vi "D-Lockin.vi"(8 "error in (no error)":errorcluster, 9 "index":u32, 10 "Stop?":bool, 11 "SweepControl":refnum<class "SMO.SweepControl.lvclass">) -> (0 "error out":errorcluster, 3 "SweepControl":refnum<class "SMO.SweepControl.lvclass">)   [LabVIEW 2019, in "SMO.SweepControl.lvclass"]
uses:
  SMO.SweepControl.lvclass
  <userlib>/LevyLab/Lockin-Multichannel/Instrument.Lockin/Instrument.Lockin.lvclass
  SMO.Transport/SMO.Transport.lvclass
  Control Experiment/Control Experiment.lvclass
  <userlib>/LevyLab/Lockin-Multichannel/Instrument.Lockin/Typedefs/Results Type--Enum.ctl
  SMO.Control Experiment/SMO.Control Experiment.lvclass
  C:/Program Files (x86)/National Instruments/LabVIEW 2019/user.lib/LevyLab/Instrument Framework/SMOs/Instrument/Instrument.lvclass
  C:/Program Files (x86)/National Instruments/LabVIEW 2019/vi.lib/JKI/JKI SMO/SMO/SMO.lvclass
panel:
  out "G4T":cluster{dbl[], dbl[]}[](graph)
  out "Y Lockins":cluster{dbl[], dbl[]}[](graph)
  out "X Lockins":cluster{dbl[], dbl[]}[](graph)
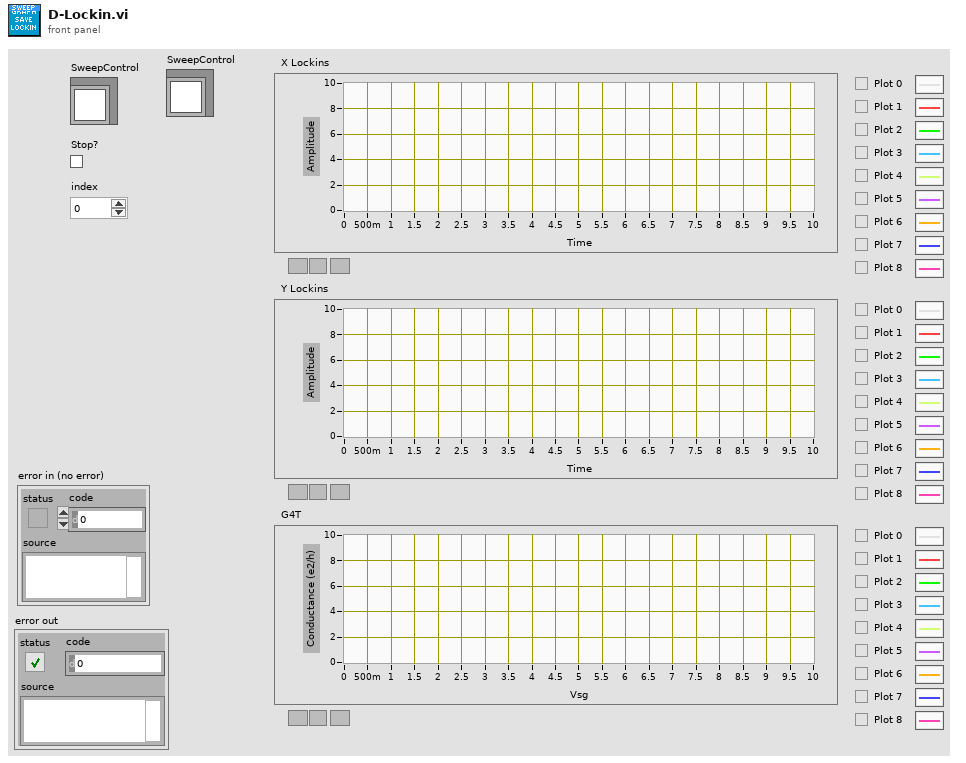
[diagram p1: front panel]
types:
  T1 = cluster{"Result X":dbl[], "Result Y":dbl[], "Data":cluster{"Y  Array":dbl[]}[], "wavenames":string[], "All Result X":dbl[][], "All Result Y":dbl[][]}
  T2 = cluster{"SweepControl":refnum<class "SMO.SweepControl.lvclass">, "data":cluster{"Result X":dbl[], "Result Y":dbl[], "Data":cluster{"Y  Array":dbl[]}[], "wavenames":string[], "All Result X":dbl[][], "All Result Y":dbl[][]}, "All Parameters":dbl[]}
  T3 = typedef "Instrument.Lockin.lvclass/Results Type--Enum.ctl" = enum16{"X", "Y", "R", "Theta", "Mean"}
  T4 = typedef "Control Experiment.lvclass/Instruments--cluster.ctl" = cluster{"KH7008":refnum<class "Instrument.KH7008.lvclass">[], "Lockin":refnum<class "Instrument.Lockin.lvclass">, "Temperature":refnum<class "Instrument.Cryostat.lvclass">, "Magnet":refnum<class "Instrument.Cryostat.lvclass">, "Rotator":refnum<class "Instrument.Cryostat.lvclass">, "Level":refnum<class "Instrument.Cryostat.lvclass">, "Capacitance Bridge":refnum<class "Instrument.CBridge.lvclass">, "Delay Line":refnum<class "Instrument.DelayLine.lvclass">, "Strain Cell":refnum<class "Instrument.Strain.lvclass">, "VNA":refnum<class "Instrument.VNA.lvclass">, "Voltage Source":refnum<class "Instrument.VSource.lvclass">}
  T5 = cluster{"I-":i32, "I+":i32, "V1-":i32, "V1+":i32, "I2-":i32, "I2+":i32, "V2-":i32, "V2+":i32}
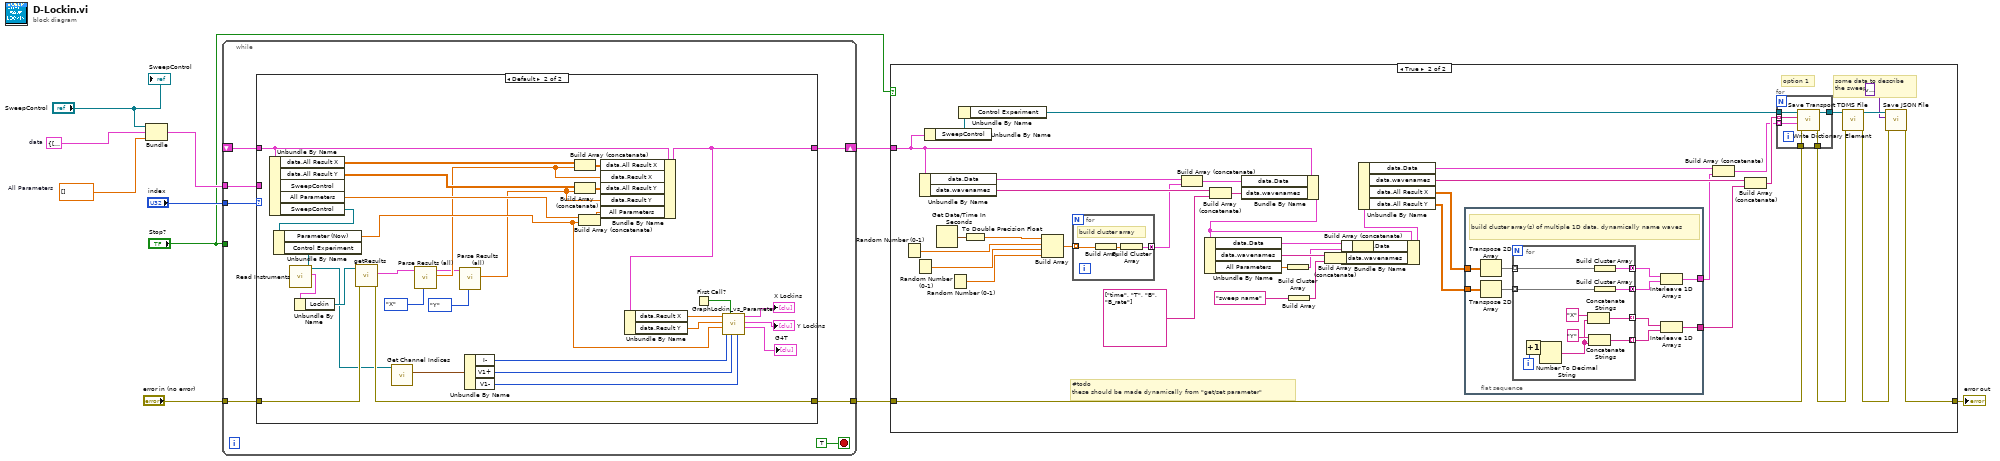
[diagram p0: block diagram]
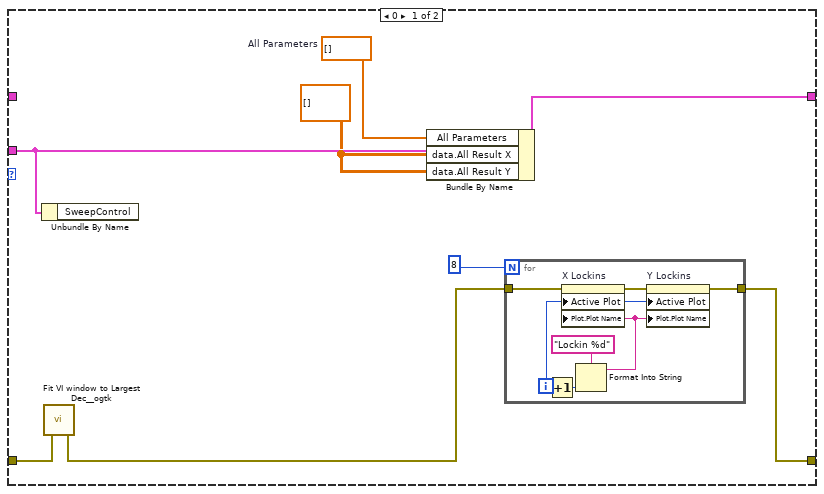
[diagram p3: hidden frame]
diagram:
  w3 = dbl[] []  # All Parameters
  w6 = T1 {"Result X"=[], "Result Y"=[], "Data"=[], "wavenames"=[], "All Result X"=[], "All Result Y"=[]}  # data
  n1 = Bundle("SweepControl"="SweepControl", "data"=w6, "All Parameters"=w3) -> (w7:T2)  [unwired: 1 in]
  n2 = while {
    tunnel: "index" -> [w17]
    tunnel: "Stop?" -> [_]
    tunnel: "error in (no error)" -> [w16]
    shift-right: [w14] -> w4
    shift-left: _ -> [w15]
    tunnel: w7 -> [w13]
    tunnel: [w12] -> w2
    stop <- TRUE stop-if-true
    n3 = case shown="Default" w17 {
      tunnel: w16 -> [w21 w60]
      tunnel: w15 -> [_ w58]
      tunnel: [w25 w56] -> w14
      tunnel: w13 -> [w24 _]
      tunnel: [w22 w59] -> w12
      frame 0 {
        w19 = dbl[] []  # All Parameters
        w20 = dbl[][] [] ("data.All Result X")
        n4 = Unbundle By Name(w24) -> ()  [unwired: 1 out]
        n5 = call <userlib>:"Fit VI window to Largest Dec__ogtk.vi"("error in (no error)"=w21) -> ("error out"=w18:errorcluster)  [unwired: 5 in, 1 out]
        n6 = Bundle By Name(cluster=w24, "All Parameters"=w19, "data.All Result X"=w20, "data.All Result Y"=w20) -> (w25:T2)
        n7 = for {
          N: 8 -> [_]
          tunnel: [w27] -> w22
          tunnel: w18 -> [w26]
          i -> [w30]
          n8 = Increment(x=w30) -> (x+1=w28:i32)
          n9 = Format Into String(format string="Lockin %d", w28) -> (resulting string=w31:string)  [unwired: 2 in, 1 out]
          n10 = property on="X Lockins" class="XYGraph (strict)"(error in=w26, "Active Plot"=w30, "Plot.Plot Name"=w31) -> (error out=w29:errorcluster)  [unwired: 1 in, 1 out]
          n11 = property on="Y Lockins" class="XYGraph (strict)"(error in=w29, "Active Plot"=w30, "Plot.Plot Name"=w31) -> (error out=w27:errorcluster)  [unwired: 1 in, 1 out]
        }
      }
      frame Default {
        n12 = Unbundle By Name(w58) -> ("data.All Result X"=w64:dbl[][], "data.All Result Y"=w63:dbl[][], "All Parameters"=w53:dbl[], "SweepControl"=w52:refnum<class "SMO.SweepControl.lvclass">)  [unwired: 1 out]
        n13 = Unbundle By Name(w52) -> ("Parameter (Now)"=w51:dbl, "Control Experiment"=w46:refnum<class "SMO.Control Experiment.lvclass">)
        n14 = call "Read Instruments.vi"("Control Experiment in"=w46) -> ("Instruments"=w45:T4, "Control Experiment out"=w43:refnum<class "Control Experiment.lvclass">)  [unwired: 8 in, 1 out]
        n15 = Unbundle By Name(w45) -> ("Lockin"=w44:refnum<class "Instrument.Lockin.lvclass">)
        n16 = call <userlib>:"getResults.vi"("error in (no error)"=w60, "Instrument.Lockin in"=w44) -> ("error out"=w59:errorcluster, "Results (Dictionary)"=w38:cluster{"key":string, "value":dbl}[])  [unwired: 6 in, 2 out]
        n17 = call "Get Channel Indices.vi"("Control Experiment in"=w43) -> ("Indices"=w42:T5)  [unwired: 8 in, 2 out]
        n18 = call <userlib>:"Parse Results (all).vi"("Type"=Results_Type--Enum."X", "Results (Dictionary)"=w38) -> ("Data"=w37:dbl[], "Results (Dictionary)"=w35:cluster{"key":string, "value":dbl}[])  [unwired: 6 in, 2 out]
        n19 = call <userlib>:"Parse Results (all).vi"("Type"=Results_Type--Enum."Y", "Results (Dictionary)"=w35) -> ("Data"=w36:dbl[])  [unwired: 6 in, 3 out]
        n20 = Unbundle By Name(w42) -> ("I-"=w41:i32, "V1+"=w40:i32, "V1-"=w39:i32)
        n21 = Build Array (concatenate)(w64, w37) -> (w61:dbl[][])
        n22 = Build Array (concatenate)(w63, w36) -> (w62:dbl[][])
        n23 = Build Array (concatenate)(w53, w51) -> (w50:dbl[])
        n24 = Bundle By Name(cluster=w58, "data.All Result X"=w61, "data.Result X"=w37, "data.All Result Y"=w62, "data.Result Y"=w36, "All Parameters"=w50) -> (w56:T2)
        n25 = Unbundle By Name(w56) -> ("data.Result X"=w57:dbl[], "data.Result Y"=w54:dbl[])
        n26 = First Call?() -> (First Call?: T/F=w55:bool)
        n27 = call "GraphLockin_vs_Parameter.vi"("V-"=w39, "V+"=w40, "reset?"=w55, "Current"=w41, "Parameter"=w51, "Y[ ]"=w54, "X[ ]"=w57) -> ("G(e2/h) vs Parameter"=→"G4T":cluster{"Y":dbl[], "Y":dbl[]}[], "Y vs Parameter"=→"Y Lockins":cluster{dbl[], dbl[]}[], "X vs Parameter"=→"X Lockins":cluster{dbl[], dbl[]}[])  [unwired: 1 in, 1 out]
      }
    }
  }
  n28 = case shown="True" "Stop?" {
    tunnel: w4 -> [_ w79]
    tunnel: w2 -> [w65 w67]
    tunnel: [w65 w73] -> w1
    frame False {
    }
    frame True {
      # "option 1"
      # "some data to describe\nthe sweep"
      # "#todo\nthese should be made dynamically from \"get/set parameter\""
      n29 = Random Number (0-1)() -> (number: 0 to 1=w96:dbl)
      n30 = Random Number (0-1)() -> (number: 0 to 1=w95:dbl)
      n31 = Unbundle By Name(w79) -> ("data.Data"=w105:cluster{"Y  Array":dbl[]}[], "data.wavenames"=w104:string[])
      n32 = Unbundle By Name(w79) -> ("SweepControl"=w78:refnum<class "SMO.SweepControl.lvclass">)
      n33 = Get Date/Time In Seconds() -> (seconds since 1Jan1904=w100:timestamp)
      n34 = Random Number (0-1)() -> (number: 0 to 1=w94:dbl)
      n35 = Unbundle By Name(w78) -> ("Control Experiment"=w68:refnum<class "SMO.Control Experiment.lvclass">)
      n36 = To Double Precision Float(number=w100) -> (double precision float=w99:dbl)
      n37 = Build Array(w99, w96, w95, w94) -> (w97:dbl[])
      n38 = for {
        tunnel: [w134] -> w98 mode=concatenating
        tunnel: w97 -> [w133] mode=indexing
        # "build cluster array"
        n39 = Build Array(w133) -> (w135:dbl[])
        n40 = Build Cluster Array(w135) -> (w134:cluster{dbl[]}[])
      }
      n41 = Build Array (concatenate)(w105, w98) -> (w102:cluster{"Y  Array":dbl[]}[])
      n42 = Build Array (concatenate)(w104, string[] ["time", "T", "B", "B_rate"] ("wavenames (.Vx, etc)")) -> (w103:string[])
      n43 = Bundle By Name(cluster=w79, "data.Data"=w102, "data.wavenames"=w103) -> (w81:T2)
      n44 = Unbundle By Name(w81) -> ("data.Data"=w93:cluster{"Y  Array":dbl[]}[], "data.wavenames"=w92:string[], "All Parameters"=w90:dbl[])
      n45 = Build Cluster Array(w90) -> (w89:cluster{"All Parameters":dbl[]}[])
      n46 = Build Array("sweep name" ("wavenames")) -> (w86:string[])
      n47 = Build Array (concatenate)(w92, w86) -> (w88:string[])
      n48 = Build Array (concatenate)(w93, w89) -> (w91:cluster{"All Parameters":dbl[]}[])
      n49 = Bundle By Name(cluster=w81, "data.Data"=w91, "data.wavenames"=w88) -> (w80:T2)
      n50 = Unbundle By Name(w80) -> ("data.Data"=w85:cluster{"Y  Array":dbl[]}[], "data.wavenames"=w84:string[], "data.All Result X"=w83:dbl[][], "data.All Result Y"=w82:dbl[][])
      n51 = flat-sequence {
        tunnel: w83 -> [w121]
        tunnel: w82 -> [w120]
        tunnel: [w113] -> w77
        tunnel: [w112] -> w76
        frame #0 {
          # "build cluster array(s) of multiple 1D data, dynamically name waves"
          n52 = Transpose 2D Array(2D array=w121) -> (transposed array=w119:dbl[][])
          n53 = Transpose 2D Array(2D array=w120) -> (transposed array=w118:dbl[][])
          n54 = for {
            tunnel: w119 -> [w132] mode=indexing
            tunnel: w118 -> [w131] mode=indexing
            tunnel: [w130] -> w117 mode=concatenating
            tunnel: [w129] -> w116 mode=concatenating
            tunnel: [w124] -> w115 mode=indexing
            tunnel: [w123] -> w114 mode=indexing
            i -> [w126]
            n55 = Increment(x=w126) -> (x+1=w122:i32)
            n56 = Number To Decimal String(number=w122) -> (decimal integer string=w125:string)  [unwired: 1 in]
            n57 = Concatenate Strings("X" ("wavenames"), w125) -> (w124:string)
            n58 = Concatenate Strings("Y" ("wavenames"), w125) -> (w123:string)
            n59 = Build Cluster Array(w132) -> (w130:cluster{dbl[]}[])
            n60 = Build Cluster Array(w131) -> (w129:cluster{dbl[]}[])
          }
          n61 = Interleave 1D Arrays(w117, w116) -> (w112:cluster{dbl[]}[])
          n62 = Interleave 1D Arrays(w115, w114) -> (w113:string[])
        }
      }
      n63 = Build Array (concatenate)(w85, w76) -> (w69:cluster{"Y  Array":dbl[]}[])
      n64 = Build Array (concatenate)(w84, w77) -> (w70:string[])
      n65 = for {
        tunnel: [w111] -> w71
        tunnel: w70 -> [w110] mode=indexing
        tunnel: w69 -> [w109] mode=indexing
        tunnel: w68 -> [w108]
        tunnel: w67 -> [w107]
        tunnel: [w106] -> w66
        n66 = call "Write Dictionary Element.vi"("error in (no error)"=w107, "value"=w109, "key"=w110, "Control Experiment in"=w108) -> ("error out"=w106:errorcluster, "Control Experiment out"=w111:refnum<class "Control Experiment.lvclass">)  [unwired: 6 in]
      }
      n67 = call "Save Transport TDMS File.vi"("error in (no error)"=w66, "Control Experiment in"=w71) -> ("error out"=w75:errorcluster, "Control Experiment out"=w74:refnum<class "Control Experiment.lvclass">)  [unwired: 8 in]
      n68 = call "Save JSON File.vi"("error in (no error)"=w75, "Data"=variant, "Control Experiment in"=w74) -> ("error out"=w73:errorcluster)  [unwired: 8 in]
    }
  }
  "error out" <- w1
  "SweepControl" <- "SweepControl"
